vi "Generate-Sound-PC-Out.vi"() -> ()   [LabVIEW 2022 SP3]
doc: "This VI illustrates how to generate and play sine, square, sawtooth and triangle waveforms. You can change the frequency and type of the waveform generated as it plays continuously."
uses:
  <vilib>/sound2/lvsound2.llb/Sampling Mode.ctl
  <vilib>/sound2/lvsound2.llb/Sound Data Format.ctl
  <vilib>/Analysis/4window.llb/windowTd.ctl
  <vilib>/sound2/lvsound2.llb/Sound Output Set Volume (Single).vi
  <vilib>/measure/matone.llb/Extract Single Tone Information 1 Chan.vi
  <vilib>/measure/maspectr.llb/FFT Spectrum (Mag-Phase) for 1 Chan.vi
  <vilib>/sound2/lvsound2.llb/Sound Output Write (DBL Single).vi
  <vilib>/measure/NI_MAPro.lvlib
  <vilib>/Analysis/NI_AALPro.lvlib
  <vilib>/measure/NI_MABase.lvlib
panel:
  out "detected frequency 2":dbl format="%.2p"
  out "detected amplitude 2":dbl format="%.2p"
  in  "Frequency":dbl=100.0
  in  "Stop 2":bool
  out "Generated Sound 2":waveform(dbl)(graph)
  in  "Volume 2":dbl(slide)=50.0 scale=0.0..100.0
  out "FFT 2":cluster{"f0":dbl, "df":dbl, "magnitude":dbl[]}(graph)
  out "detected amplitude":dbl format="%.2p"
  out "detected frequency":dbl format="%.2p"
  out "FFT":cluster{"f0":dbl, "df":dbl, "magnitude":dbl[]}(graph)
  in  "Volume":dbl(slide)=50.0 scale=0.0..100.0
  out "Generated Sound":waveform(dbl)(graph)
  in  "Standard Deviation":dbl=1.0
  in  "Stop":bool
  in  "Device ID":u32
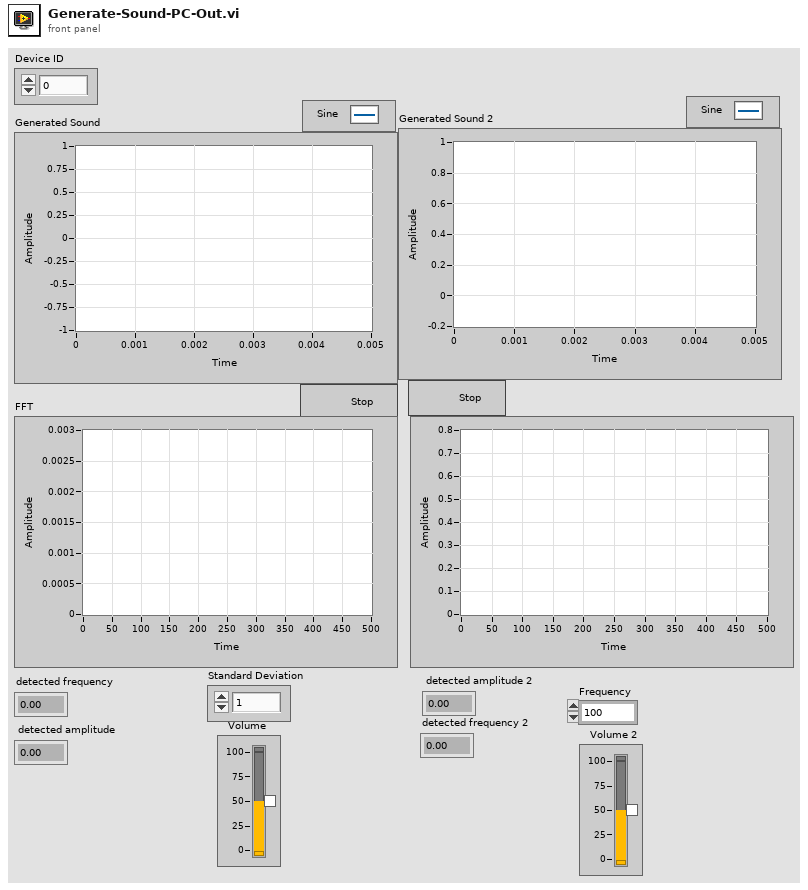
[diagram p1: front panel]
types:
  T1 = typedef "Sound Data Format.ctl" = cluster{"sample rate (S/s)":dbl, "number of channels":i32, "bits per sample":i32}
  T2 = typedef "Sampling Mode.ctl" = i32
  T3 = typedef "Sound Output Task ID.ctl" = u32
  T4 = cluster{"averaging mode":enum16{"No averaging", "Vector averaging", "RMS averaging", "Peak hold"}, "weighting mode":enum16{"Linear", "Exponential"}, "number of averages":u32}
  T5 = cluster{"dB On (F)":bool, "unwrap phase (F)":bool, "convert to degree (F)":bool}
  T6 = typedef "NI_AALPro.lvlib/windowTd.ctl" = u32
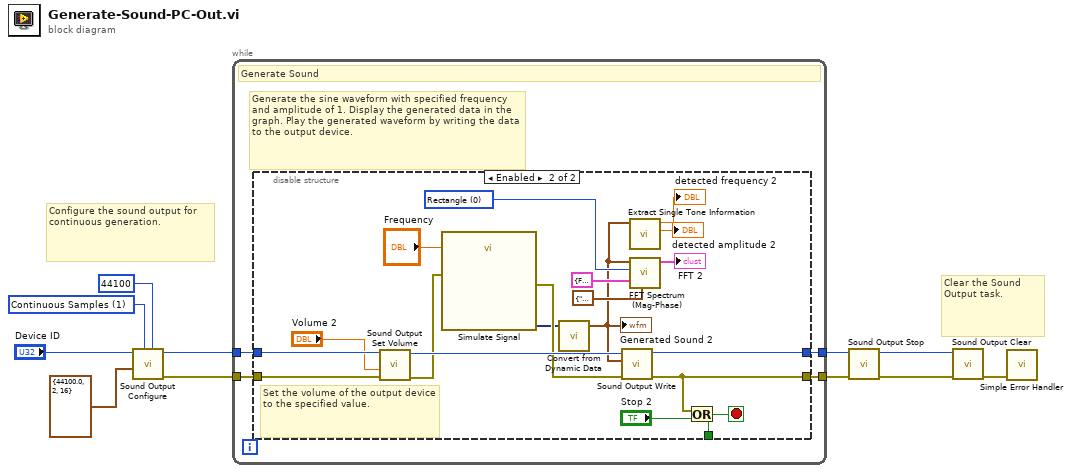
[diagram p0: block diagram]
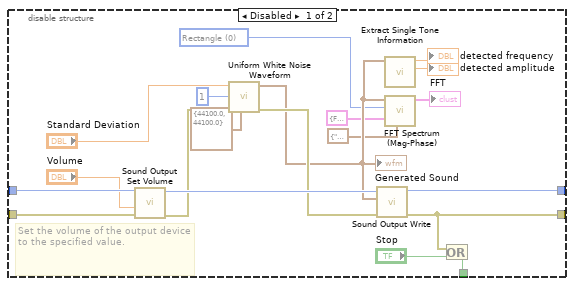
[diagram p2: hidden frame]
diagram:
  w7 = T2 1 items=["Finite Samples", "Continuous Samples"] ("sample mode")
  # "Configure the sound output for continuous generation."
  # "Clear the Sound Output task."
  n1 = call <vilib>:"Sound Output Configure.vi"("number of samples/ch"=44100 ("Number of Samples/ch"), "sample mode"=w7, "sound format"=T1 {"sample rate (S/s)"=44100.0, "number of channels"=2, "bits per sample"=16} ("Sound Format"), "device ID"="Device ID") -> ("error out"=w11:errorcluster, "task ID"=w10:T3)  [unwired: 6 in]
  n2 = while {
    tunnel: w10 -> [w13]
    tunnel: [w16] -> w9
    tunnel: w11 -> [w14]
    tunnel: [w12] -> w2
    stop <- w15 stop-if-true
    # "Generate the sine waveform with specified frequency and amplitude of 1. Display the generated data in the graph. Play the generated waveform by writing the data to the output device."
    # "Generate Sound"
    n3 = disable-structure shown="Enabled" {
      disable-tunnel: [w36 w55] -> w16
      disable-tunnel: [w34 w53] -> w15
      disable-tunnel: w14 -> [w33 w52]
      disable-tunnel: w13 -> [w31 w50]
      disable-tunnel: [w29 w48] -> w12
      frame Disabled {
        w20 = T6 0 items=["Rectangle"=0, "Hanning"=1, "Hamming"=2, "Blackman-Harris"=3, "Exact Blackman"=4, "Blackman"=5, "Flat Top"=6, "4 Term B-Harris "=7, "7 Term B-Harris"=8, "Low Sidelobe"=9, "Blackman Nuttall"=11, "Triangle"=30, "Bartlett-Hanning"=31, "Bohman"=32, "Parzen"=33, "Welch"=34, "Kaiser"=60, "Dolph-Chebyshev"=61, "Gaussian"=62] ("window")
        # "Set the volume of the output device to the specified value."
        n4 = call-poly <vilib>:"Sound Output Set Volume.vi"("error in (no error)"=w33, "volume"="Volume", "task ID"=w31) -> ("error out"=w28:errorcluster, "task ID out"=w32:T3)  [unwired: 7 in]
        n5 = call <vilib>:"Uniform White Noise Waveform.vi"("sampling info"=cluster{"Fs":dbl, "#s":dbl} {"Fs"=44100.0, "#s"=44100.0}, "error in (no error)"=w28, "seed"=1, "amplitude"="Standard Deviation") -> ("error out"=w27:errorcluster, "signal out"=w23:waveform(dbl))  [unwired: 6 in]
        "Generated Sound" <- w23
        n6 = call-poly <vilib>:"Sound Output Write.vi"("error in (no error)"=w27, "data"=w23, "task ID"=w32) -> ("error out"=w29:errorcluster, "task ID out"=w36:T3)  [unwired: 7 in]
        n7 = call-poly <vilib>:"Extract Single Tone Information.vi"("time signal in"=w23) -> ("detected amplitude"=→"detected amplitude":dbl, "detected frequency"=→"detected frequency":dbl)  [unwired: 5 in, 4 out]
        n8 = call-poly <vilib>:"FFT Spectrum (Mag-Phase).vi"("averaging parameters"=T4 {"averaging mode"=enum."Vector averaging", "weighting mode"=enum."Linear", "number of averages"=10}, "view"=T5 {"dB On (F)"=FALSE, "unwrap phase (F)"=FALSE, "convert to degree (F)"=FALSE}, "window"=w20, "time signal"=w23) -> ("magnitude"=→"FFT":cluster{"f0":dbl, "df":dbl, "magnitude":dbl[]})  [unwired: 3 in, 4 out]
        n9 = Or(x=w29, y="Stop") -> (x .or. y?=w34:bool)
      }
      frame Enabled {
        w43 = T6 0 items=["Rectangle"=0, "Hanning"=1, "Hamming"=2, "Blackman-Harris"=3, "Exact Blackman"=4, "Blackman"=5, "Flat Top"=6, "4 Term B-Harris "=7, "7 Term B-Harris"=8, "Low Sidelobe"=9, "Blackman Nuttall"=11, "Triangle"=30, "Bartlett-Hanning"=31, "Bohman"=32, "Parzen"=33, "Welch"=34, "Kaiser"=60, "Dolph-Chebyshev"=61, "Gaussian"=62] ("window")
        # "Set the volume of the output device to the specified value."
        n10 = call-poly <vilib>:"Sound Output Set Volume.vi"("error in (no error)"=w52, "volume"="Volume 2", "task ID"=w50) -> ("error out"=w47:errorcluster, "task ID out"=w51:T3)  [unwired: 7 in]
        n11 = call "Simulate Signal"("Frequency"="Frequency", "error in (no error)"=w47) -> ("Sine"=w44:dynamicdata, "error out"=w46:errorcluster)  [unwired: 12 in]
        n12 = call "Convert from Dynamic Data"("Dynamic Data Type"=w44) -> ("Waveform"=w40:waveform(dbl))  [unwired: 3 in]
        "Generated Sound 2" <- w40
        n13 = call-poly <vilib>:"Sound Output Write.vi"("error in (no error)"=w46, "data"=w40, "task ID"=w51) -> ("error out"=w48:errorcluster, "task ID out"=w55:T3)  [unwired: 7 in]
        n14 = call-poly <vilib>:"Extract Single Tone Information.vi"("time signal in"=w40) -> ("detected amplitude"=→"detected amplitude 2":dbl, "detected frequency"=→"detected frequency 2":dbl)  [unwired: 5 in, 4 out]
        n15 = call-poly <vilib>:"FFT Spectrum (Mag-Phase).vi"("averaging parameters"=T4 {"averaging mode"=enum."Vector averaging", "weighting mode"=enum."Linear", "number of averages"=10}, "view"=T5 {"dB On (F)"=FALSE, "unwrap phase (F)"=FALSE, "convert to degree (F)"=FALSE}, "window"=w43, "time signal"=w40) -> ("magnitude"=→"FFT 2":cluster{"f0":dbl, "df":dbl, "magnitude":dbl[]})  [unwired: 3 in, 4 out]
        n16 = Or(x=w48, y="Stop 2") -> (x .or. y?=w53:bool)
      }
    }
  }
  n17 = call <vilib>:"Sound Output Stop.vi"("error in (no error)"=w2, "task ID"=w9) -> ("error out"=w1:errorcluster, "task ID out"=w3:T3)  [unwired: 8 in]
  n18 = call <vilib>:"Sound Output Clear.vi"("error in (no error)"=w1, "task ID"=w3) -> ("error out"=w5:errorcluster)  [unwired: 9 in]
  n19 = call <vilib>:"Simple Error Handler.vi"("error in (no error)"=w5) -> ()  [unwired: 4 in, 5 out]
